vi "Launch ManualUI.vi"(8 "error in (no error)":errorcluster, 11 "Main in":refnum<class "Main.lvclass">) -> (0 "error out":errorcluster, 3 "Main out":refnum<class "Main.lvclass">)   [LabVIEW 2023, in "Main.lvlib" / "Main.lvclass"]
uses:
  Library/Main.lvclass
  Library/Main.lvclass/Main.ctl
  builds/Framework/Engine.lvlibp/Managed Actor/Library/Managed Actor.lvclass
  builds/Framework/Engine.lvlibp/Engine/Library/Engine.lvclass
  C:/Users/Public/Documents/Development/builds/Framework/Engine.lvlibp/Managed Actor/Library/Managed Actor.lvclass
  C:/Users/Public/Documents/Development/builds/Framework/Engine.lvlibp/Engine/Library/Engine.lvclass
  C:/Users/Public/Documents/Development/builds/Framework/Panel Manager.lvlibp/Library/Panel Actor.lvclass
  C:/Users/Public/Documents/Development/builds/Framework/Monitored Actor.lvlibp/Actor Monitor/Actor Monitor/Actor Monitor.lvclass
  C:/Users/Public/Documents/Development/builds/Framework/Actor Framework.lvlibp/1abvi3w/vi.lib/ActorFramework/Actor/Actor.lvclass
  C:/Users/Public/Documents/Development/Application/Main/Library/Main.lvclass
  builds/Main/Docking.lvlibp/Docking/Docking.lvclass
  Custom Controls/Components.vi
  builds/Main/ManualUI.lvlibp/Library/ManualUI.lvclass
  C:/Users/Public/Documents/Development/builds/Main/Docking.lvlibp/Prime Panel/PrimeDock.lvclass
  C:/Users/Public/Documents/Development/builds/Main/Docking.lvlibp/Docking/Docking.lvclass
  C:/Users/Public/Documents/Development/builds/Main/ManualUI.lvlibp/Library/ManualUI.lvclass
  builds/Framework/Panel Manager.lvlibp/Panel/Panel/Subpanel/Subpanel.lvclass
  C:/Users/Public/Documents/Development/builds/Framework/Panel Manager.lvlibp/Panel/Panel/Panel.lvclass
  C:/Users/Public/Documents/Development/builds/Framework/Panel Manager.lvlibp/Panel/Panel/Subpanel/Subpanel.lvclass
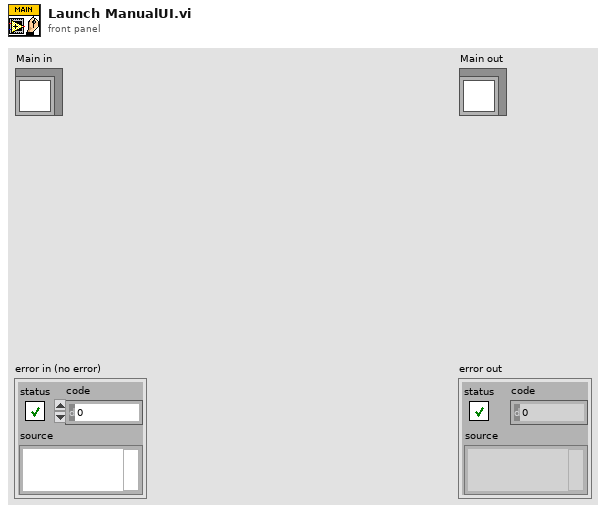
[diagram p1: front panel]
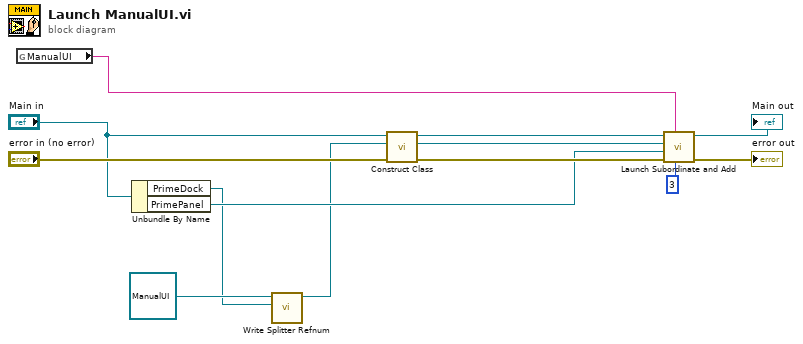
[diagram p0: block diagram]
diagram:
  n1 = global read "Components.vi" "ManualUI"() -> (w1:string)
  n2 = Unbundle By Name("Main in") -> ("PrimeDock"=w3:refnum<vi>, "PrimePanel"=w6:refnum<class "Subpanel.lvclass">)
  n3 = call "Write Splitter Refnum.vi"("Splitter Refnum"=w3, "Docking in"=refnum<class "ManualUI.lvclass"> refnum ("ManualUI.lvlibp:ManualUI.lvclass")) -> ("Docking out"=w4:refnum<class "ManualUI.lvclass">)  [unwired: 8 in, 1 out]
  n4 = call "Construct Class.vi"("error in (no error)"="error in (no error)", "Actor in"=w4, "Engine in"="Main in") -> ("error out"=w10:errorcluster, "Actor out"=w11:refnum<class "ManualUI.lvclass">, "Engine out"=w12:refnum<class "Main.lvclass">)  [unwired: 6 in]
  n5 = call "Launch Subordinate and Add.vi"("PanelIndex"=3, "Identifier"=w1, "error in (no error)"=w10, "Panel"=w6, "Nested Panel Actor"=w11, "Managed Actor in"=w12) -> ("error out"=→"error out":errorcluster, "Managed Actor out"=→"Main out":refnum<class "Main.lvclass">)  [unwired: 4 in]
